vi "测试效率.vi"() -> ()   [LabVIEW 2016]
uses:
  <vilib>/measure/NI_MABase.lvlib
  SubVIs/VCH/Private/Ctrls/PSVCH_VarList.ctl
panel:
  out "x-y":u32
  in  "Formula Node":T1={"Formula Steps"=[{"Formula Calc"="+", "Para"=[{"Para Index"=0, "Tag"="Var", "Type"="Analog Waveform", "Label"="a0", "Data"=variant}, {"Para Index"=-1, "Tag"="3", "Type"="Dbl", "Label"="3", "Data"=variant(dbl 3.0)}], "Result Var"="Var0", "Result Var Type"="Analog Waveform"}], "MidVar List"={"Names"=["Var0"], "Types"=["Analog Waveform"], "Values"=[variant(waveform(dbl) {"t0"=timestamp(0 s since 1904-01-01), "dt"=0.0, "Y"=[]})]}}
  in  "VarList":T2={"Tag[]"=["CH1"], "Type[]"=["Waveform"], "Value[]"=[variant(waveform(dbl) {"t0"=timestamp(0 s since 1904-01-01), "dt"=0.0, "Y"=[]})], "ai[]"=["a0"]}
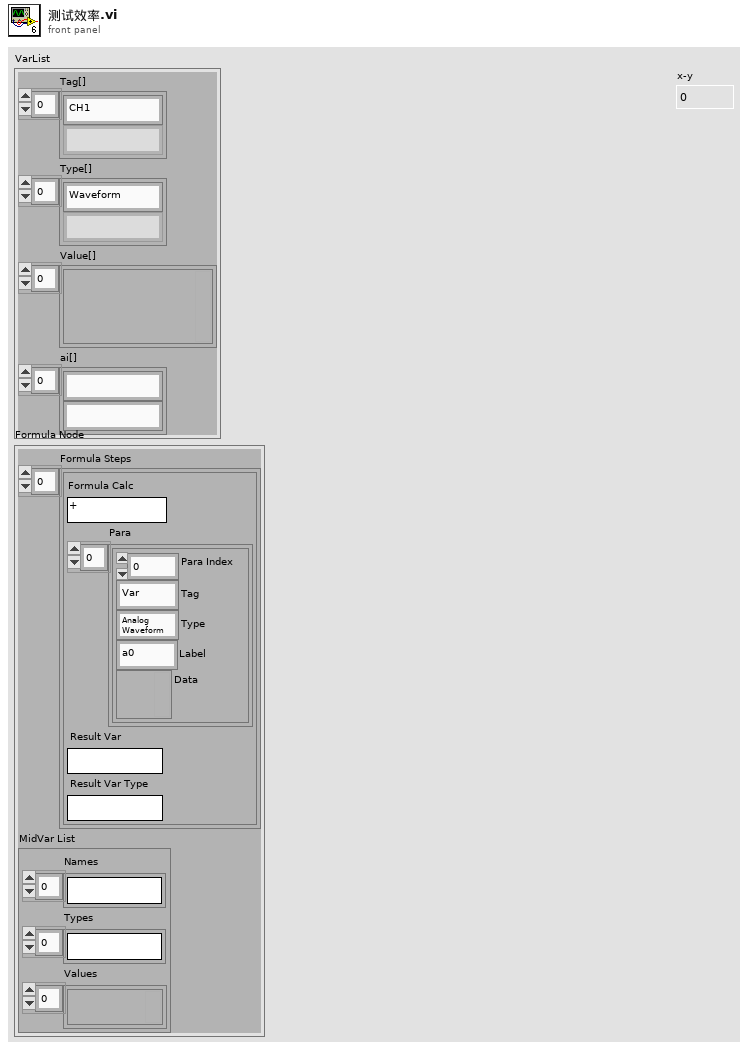
[diagram p1: front panel]
types:
  T1 = cluster{"Formula Steps":cluster{"Formula Calc":string, "Para":cluster{"Para Index":i32, "Tag":string, "Type":string, "Label":string, "Data":variant}[], "Result Var":string, "Result Var Type":string}[], "MidVar List":cluster{"Names":string[], "Types":string[], "Values":variant[]}}
  T2 = typedef "PSVCH_VarList.ctl" = cluster{"Tag[]":string[], "Type[]":string[], "Value[]":variant[], "ai[]":string[]}
  T3 = cluster{"ai[]":string[], "Type[]":string[], "Value[]":variant[]}
  T4 = cluster{"Name":string, "Type":string, "Value":variant}
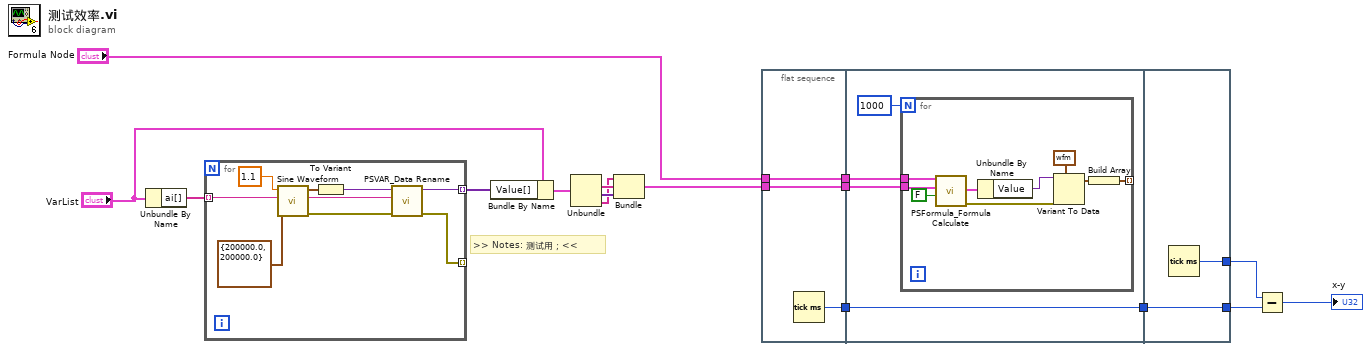
[diagram p0: block diagram]
diagram:
  # ">> Notes: 测试用；<<"
  n1 = Unbundle By Name("VarList") -> ("ai[]"=w13:string[])
  n2 = for {
    tunnel: [w19] -> _ mode=indexing
    tunnel: w13 -> [w18] mode=indexing
    tunnel: [w17] -> w12 mode=indexing
    n3 = call <vilib>:"Sine Waveform.vi"("sampling info"=cluster{"Fs":dbl, "#s":dbl} {"Fs"=200000.0, "#s"=200000.0}, "frequency"=1.1) -> ("error out"=w20:errorcluster, "signal out"=w22:waveform(dbl))  [unwired: 8 in]
    n4 = To Variant(anything=w22) -> (Variant=w21:variant)
    n5 = call <vilib>:"PSVAR_Data Rename.vi"("error in"=w20, "Name New"=w18, "Data In"=w21) -> ("error out"=w19:errorcluster, "Data Out"=w17:variant)  [unwired: 7 in]
  }
  n6 = Bundle By Name(cluster="VarList", "Value[]"=w12) -> (w9:T2)
  n7 = Unbundle(w9) -> ("Type[]"=w16:string[], "Value[]"=w15:variant[], "ai[]"=w14:string[])  [unwired: 1 out]
  n8 = Bundle("ai[]"=w14, "Type[]"=w16, "Value[]"=w15) -> (w8:T3)  [unwired: 1 in]
  n9 = flat-sequence {
    tunnel: "Formula Node" -> [w26]
    tunnel: w8 -> [w27]
    tunnel: [w27] -> w7
    tunnel: [w26] -> w6
    tunnel: [w25] -> w5
    tunnel: w7 -> [w31]
    tunnel: w6 -> [w30]
    tunnel: [w28] -> w4
    tunnel: w5 -> [w28]
    tunnel: w4 -> [w42]
    tunnel: [w42] -> w3
    tunnel: [w41] -> w2
    frame #0 {
      n10 = Tick Count (ms)() -> (millisecond timer value=w25:u32)
    }
    frame #1 {
      n11 = for {
        N: 1000 -> [_]
        tunnel: w31 -> [w38]
        tunnel: w30 -> [w39]
        tunnel: [w33] -> _ mode=indexing
        n12 = call "PSFormula_Formula Calculate.vi"("Complex Variable(T)"=FALSE, "Var List"=w38, "Formula Node"=w39) -> ("error out"=w34:errorcluster, "Result"=w36:T4)  [unwired: 6 in, 1 out]
        n13 = Unbundle By Name(w36) -> ("Value"=w35:variant)
        n14 = Variant To Data(error in=w34, type=waveform(dbl) {"t0"=timestamp(0 s since 1904-01-01), "dt"=1.0, "Y"=[]} ("Waveform"), Variant=w35) -> (data=w37:waveform(dbl))  [unwired: 1 out]
        n15 = Build Array(w37) -> (w33:waveform(dbl)[])
      }
    }
    frame #2 {
      n16 = Tick Count (ms)() -> (millisecond timer value=w41:u32)
    }
  }
  n17 = Subtract(x=w2, y=w3) -> (x-y=→"x-y":u32)
